vi "Packetize.vi"(8 "Error In":errorcluster, 9 "Data":u8[](array[numeric]) format="%2x", 10 "Command":T2, 11 "EZ430-Chronos Config":T1) -> (0 "Error Out":errorcluster, 2 "Packet":string, 3 "EZ430-Chronos Config":T1)   [LabVIEW 2011, in "LVH-EZ430.lvlib"]
uses:
  LVH-EZ430.lvlib
  Type Defs/Command.ctl
  Type Defs/EZ430-Chronos Ref.ctl
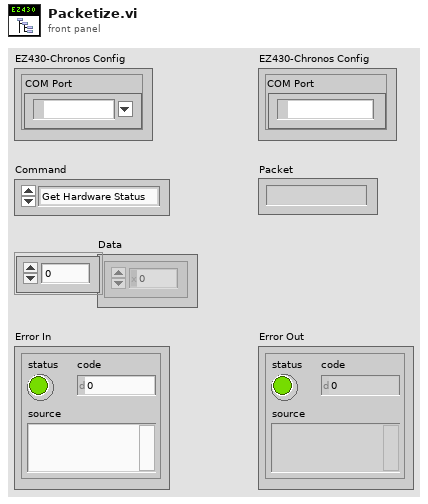
[diagram p1: front panel]
types:
  T1 = typedef "LVH-EZ430.lvlib/EZ430-Chronos Ref.ctl" = cluster{"COM Port":refnum<visa-resource-name>}
  T2 = typedef "LVH-EZ430.lvlib/Command.ctl" = enum8{"Get Hardware Status", "Reset RF Access Point", "Start BlueRobin Transmitter", "Set BlueRobin Trans ID", "Get BlueRobin Trans ID", "Set BlueRobin Heart Rate To Transmit", "Stop BlueRobin Transmitter", "Start ACC / PPT Mode", "Read ACC / PPT", "Stop SimpliciTI Stack"}
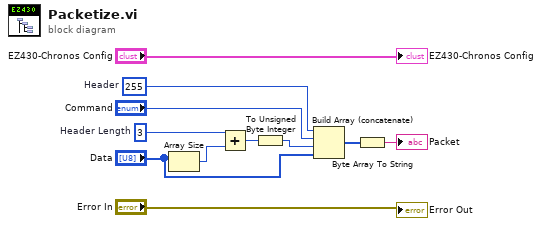
[diagram p0: block diagram]
diagram:
  w6 = 3  # Header Length
  w3 = u8 255  # Header
  n1 = Array Size(array="Data") -> (size(s)=w5:i32)
  n2 = Add(x=w6, y=w5) -> (x+y=w7:i32)
  n3 = To Unsigned Byte Integer(number=w7) -> (unsigned 8bit integer=w8:u8)
  n4 = Build Array (concatenate)(w3, "Command", w8, "Data") -> (w10:u8[])
  n5 = Byte Array To String(unsigned byte array=w10) -> (string=→"Packet":string)
  "Error Out" <- "Error In"
  "EZ430-Chronos Config" <- "EZ430-Chronos Config"
